vi "ToSettingsCluster.vi"(0 "Element Names (destination) out":string[](array[string]), 1 "variant  (source)":variant, 2 "Element Names (source)":string[](array[string]), 3 "error out":errorcluster, 4 "variant (destination)":variant) -> (5 "variant (destination) out":variant, 6 "error out 2":errorcluster)   [LabVIEW 2011]
uses:
  OnOffTypeDef.ctl
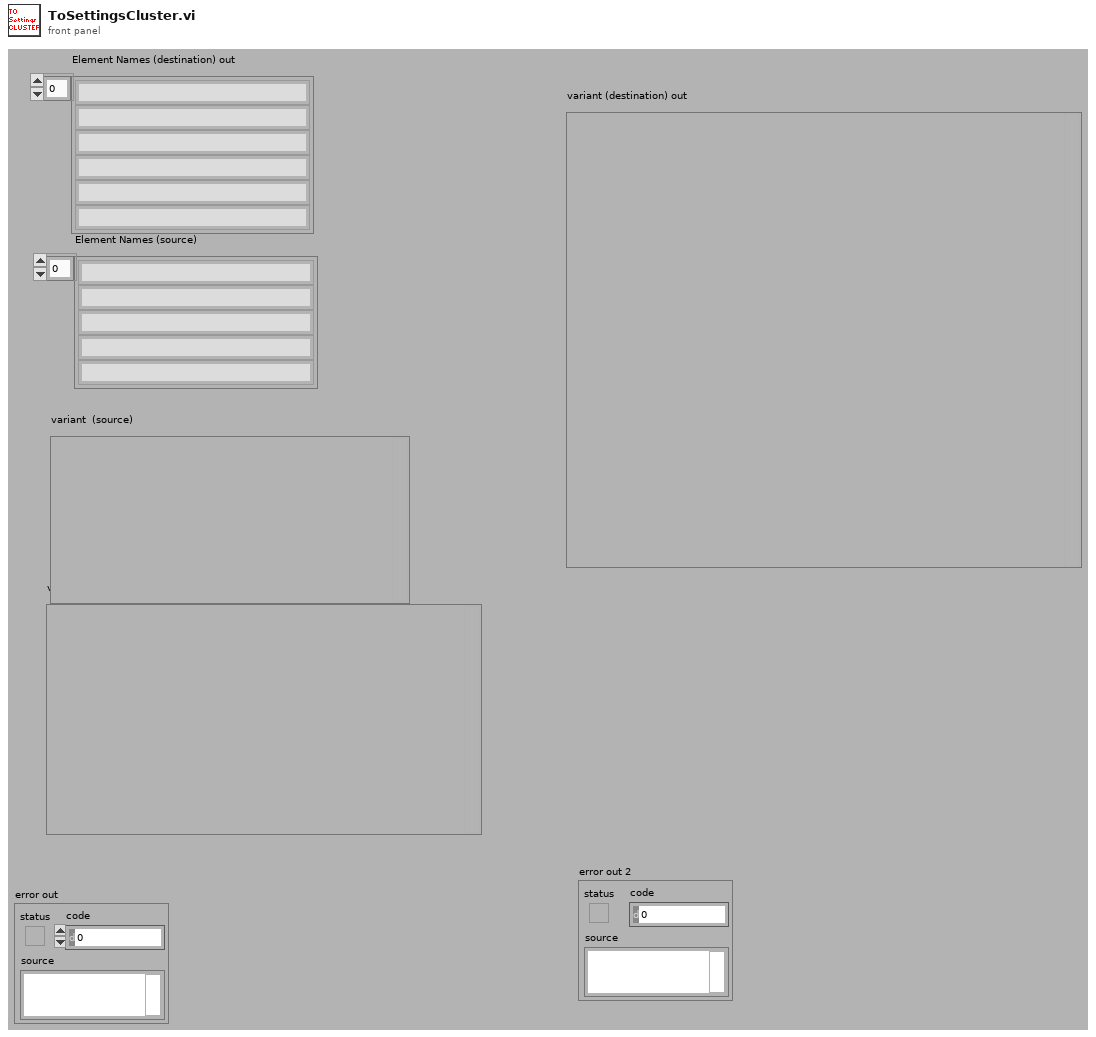
[diagram p1: front panel]
types:
  T1 = typedef "OnOffTypeDef.ctl" = enum16{"off", "on"}
  T2 = typedef "Type Descriptor Enumeration__ogtk.ctl" = enum8{"<Null>", "I8", "I16", "I32", "I64", "U8", "U16", "U32", "U64", "SGL", "DBL", "EXT", "CSG", "CDB", "CXT", "0x0F", "0x10", "0x11", "0x12", "0x13", "0x14", "Enum U8", "Enum U16", "Enum U32", "Enum U64", "SGL PQ", "DBL PQ", "EXT PQ", "CSG PQ", "CDB PQ", "CXT PQ", "0x1F", "0x20", "Boolean", "0x22", "0x23", "0x24", "0x25", "0x26", "0x27", "0x28", "0x29", "0x2A", "0x2B", "0x2C", "0x2D", "0x2E", "0x2F", "String", "0x31", "Path", "Pict", "0x34", "0x35", "0x36", "DAQ", "0x38", "0x39", "0x3A", "0x3B", "0x3C", "0x3D", "0x3E", "0x3F", "Array", "0x41", "0x42", "0x43", "0x44", "0x45", "0x46", "0x47", "0x48", "0x49", "0x4A", "0x4B", "0x4C", "0x4D", "0x4E", "0x4F", "Cluster", "0x51", "0x52", "Variant", "Waveform", "0x55", "0x56", "0x57", "0x58", "0x59", "0x5A", "0x5B", "0x5C", "0x5D", "0x5E", "0x5F", "0x60", "0x61", "0x62", "0x63", "0x64", "0x65", "0x66", "0x67", "0x68", "0x69", "0x6A", "0x6B", "0x6C", "0x6D", "0x6E", "0x6F", "Refnum"}
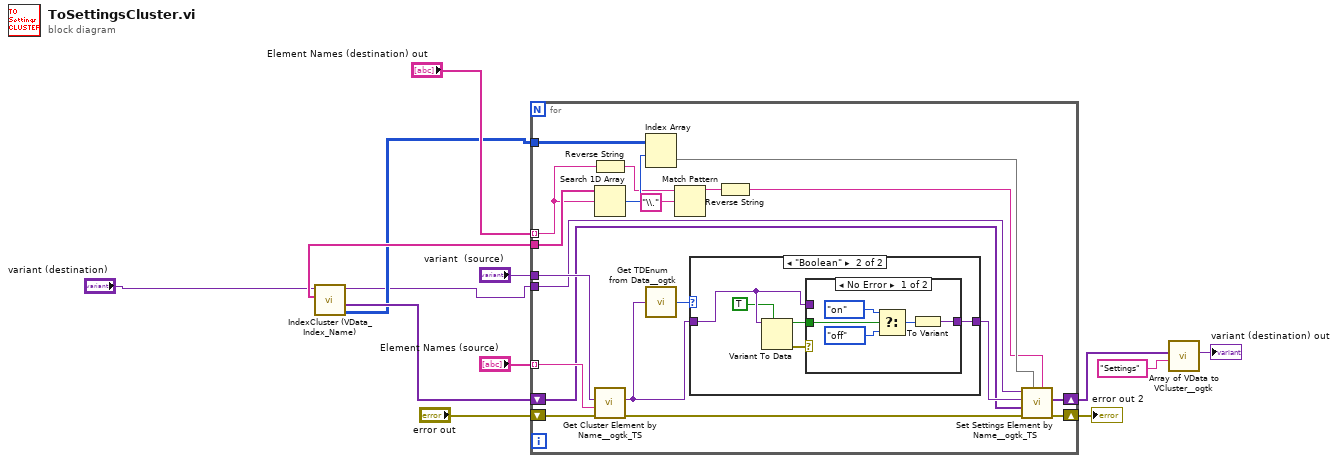
[diagram p0: block diagram]
diagram:
  n1 = call "IndexCluster (VData_Index_Name).vi"("variant (destination)"="variant (destination)") -> ("index Array"=w2:i32[][], "Array of VData"=w8:variant[], "Names (Array)"=w9:string[], "variant (destination)out"=w1:variant)  [unwired: 7 in]
  n2 = for {
    tunnel: "Element Names (source)" -> [w33] mode=indexing
    tunnel: "variant  (source)" -> [w32]
    shift-right: [w15] -> w11
    shift-left: "error out" -> [w29]
    tunnel: "Element Names (destination) out" -> [w18] mode=indexing
    shift-right: [w27] -> w6
    shift-left: w8 -> [w26]
    tunnel: w9 -> [w25]
    tunnel: w2 -> [w24]
    tunnel: w1 -> [w14]
    n3 = Reverse String(1:w18) -> (0:w21:string)
    n4 = Search 1D Array(1D array=w25, element=w18) -> (index of element=w23:i32)  [unwired: 1 in]
    n5 = call "Get Cluster Element by Name__ogtk_TS.vi"("error in (no error)"=w29, "Element Name"=w33, "Cluster"=w32) -> ("error out"=w16:errorcluster, "VElement"=w31:variant)  [unwired: 6 in, 1 out]
    n6 = Index Array(array=w24, index (row)=w23) -> (element=w22:i32[])  [unwired: 1 in]
    n7 = call "Get TDEnum from Data__ogtk.vi"("Data"=w31) -> ("Type Descriptor Enumeration"=w30:T2)  [unwired: 4 in]
    n8 = Match Pattern(string=w21, regular expression="\\.") -> (before substring=w19:string)  [unwired: 1 in, 3 out]
    n9 = case shown="\"Boolean\"" w30 {
      tunnel: [w34 w37] -> w28
      tunnel: w31 -> [w34 w36]
      frame "<Null>", Default {
      }
      frame "Boolean" {
        n10 = Variant To Data(type=TRUE, Variant=w36) -> (data=w38:bool, error out=w39:errorcluster)  [unwired: 1 in]
        n11 = case shown="No Error" w39 {
          tunnel: w38 -> [w43 _]
          tunnel: [w44 w45] -> w37
          tunnel: w36 -> [_ w45]
          frame No Error {
            n12 = Select(t=OnOffTypeDef."on" ("Save"), s=w43, f=OnOffTypeDef."off" ("Save")) -> (s? t:f=w41:T1)
            n13 = To Variant(anything=w41) -> (Variant=w44:variant)
          }
          frame Error {
          }
        }
      }
    }
    n14 = Reverse String(1:w19) -> (0:w17:string)
    n15 = call "Set Settings Element by Name__ogtk_TS.vi"("element Name"=w17, "index Array"=w22, "error in (no error)"=w16, "Settings VData"=w26, "New Element Value"=w28, "Cluster"=w14) -> ("error out"=w15:errorcluster, "Settings VData out"=w27:variant[])  [unwired: 4 in]
  }
  "error out 2" <- w11
  n16 = call "Array of VData to VCluster__ogtk.vi"("Cluster Name"="Settings" ("Data Name"), "Array"=w6) -> ("VCluster"=→"variant (destination) out":variant)  [unwired: 8 in, 1 out]
